vi "AI Channel Update.vi"(7 "Device Ref":T4 format="%.0x", 8 "error in (no error)":errorcluster caption="错误输入（无错误）", 11 "DIChannel":T1[](array[typedef])) -> (0 "error out":errorcluster caption="错误输出")   [LabVIEW 2013]
uses:
  <vilib>/K2Labs/HiLab API/Custom Device API/Controls/Custom Device Item Reference.ctl
  AI Param.ctl
  MeasurementType.ctl
  AI Terminal Configuration.ctl
  <vilib>/K2Labs/HiLab API/Custom Device API/Controls/Custom Device Channel.ctl
  <vilib>/K2Labs/HiLab API/Custom Device API/Controls/Custom Device Channel Dimensions.ctl
  <vilib>/K2Labs/HiLab API/Custom Device API/Controls/Custom Device Channel Type.ctl
  <vilib>/K2Labs/HiLab API/Custom Device API/Configuration/Item Properties/Set Item Property/Set Item Property(String).vi
  <vilib>/K2Labs/HiLab API/Custom Device API/Configuration/Item Properties/Set Item Property/Set Item Property(I16).vi
  <vilib>/K2Labs/HiLab API/Custom Device API/Configuration/Item Properties/Set Item Property/Set Item Property(Double).vi
  <vilib>/K2Labs/HiLab API/Custom Device API/Custom Device API Library.lvlib
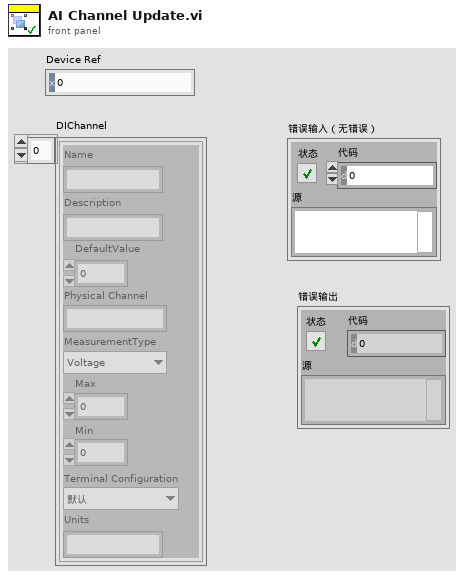
[diagram p1: front panel]
types:
  T1 = typedef "AI Param.ctl" = cluster{"Name":string, "Description":string, "DefaultValue":dbl, "Physical Channel":string, "MeasurementType":T2, "Max":dbl, "Min":dbl, "Terminal Configuration":T3, "Units":string}
  T2 = typedef "MeasurementType.ctl" = enum16{"Voltage", "Current", "More:Voltage:Custom with Excitation", "More:Current:Custom with Excitation", "Frequency", "Period", "Resistance", "Temperature:Thermocouple", "Temperature:Thermistor", "Temperature:RTD", "Temperature:Built-in Sensor", "Strain Gage"}
  T3 = typedef "AI Terminal Configuration.ctl" = enum16{"默认", "RSE", "NRSE", "差分", "伪差分"}
  T4 = typedef "Custom Device API Library.lvlib/Custom Device Item Reference.ctl" = u64
  T5 = typedef "Custom Device API Library.lvlib/Custom Device Channel.ctl" = cluster{"DefaultValue":dbl[], "Dimensions":T6, "Units":string, "Type":T7}
  T6 = typedef "Custom Device API Library.lvlib/Custom Device Channel Dimensions.ctl" = cluster{"Row":i32, "Column":i32}
  T7 = typedef "Custom Device API Library.lvlib/Custom Device Channel Type.ctl" = enum16{"Input", "Output"}
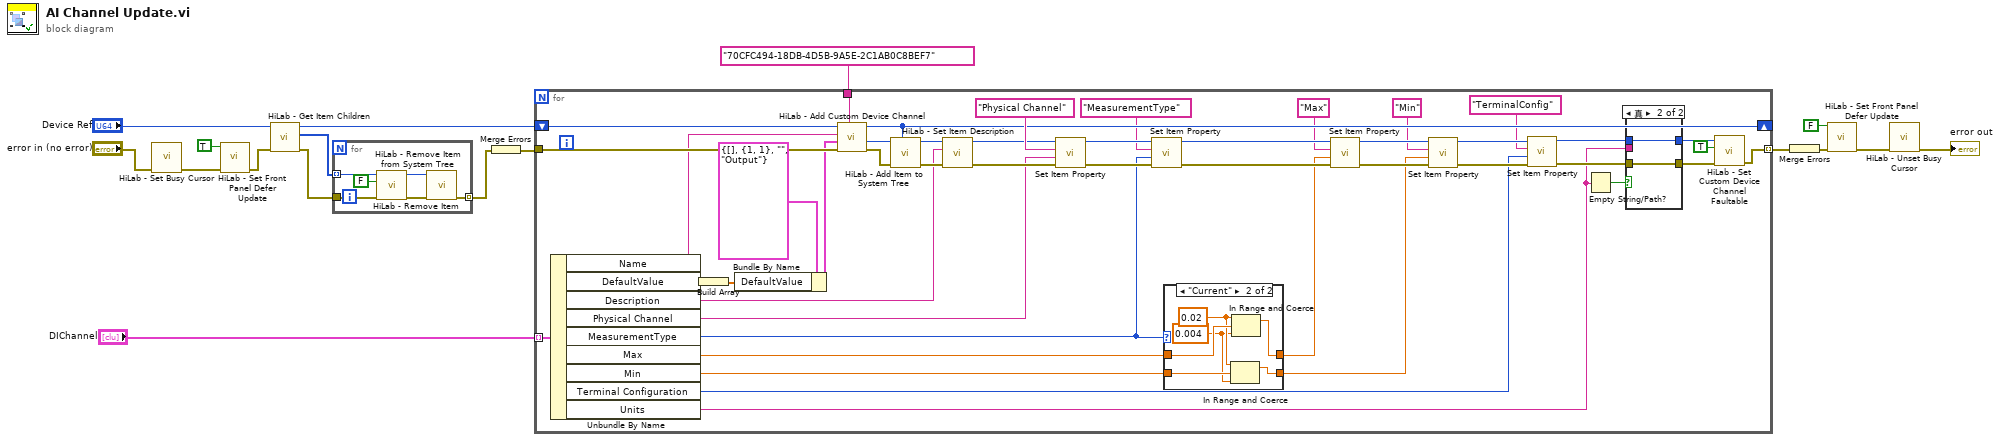
[diagram p0: block diagram]
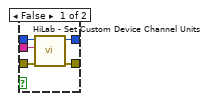
[diagram p2: hidden frame]
diagram:
  n1 = call <vilib>:"HiLab - Set Busy Cursor.vi"("error in (no error)"="error in (no error)") -> ("error out"=w15:errorcluster)  [unwired: 10 in]
  n2 = call <vilib>:"HiLab - Set Front Panel Defer Update.vi"("error in (no error)"=w15, "DeferSystemConfigurationPanUpdates(F)"=TRUE) -> ("error out"=w5:errorcluster)  [unwired: 9 in]
  n3 = call <vilib>:"HiLab - Get Item Children.vi"("error in (no error)"=w5, "Item Ref in"="Device Ref") -> ("error out"=w8:errorcluster, "Child Refs"=w7:T4[], "Item Ref out"=w3:T4)  [unwired: 6 in, 1 out]
  n4 = for {
    tunnel: w8 -> [w20]
    tunnel: [w19] -> w9 mode=indexing
    tunnel: w7 -> [w18] mode=indexing
    n5 = call <vilib>:"HiLab - Remove Item from System Tree.vi"("error in (no error)"=w20, "HighLightPreviousItem?(T)"=FALSE, "Item Ref in"=w18) -> ("error out"=w22:errorcluster, "Item Ref out"=w23:T4)  [unwired: 7 in]
    n6 = call <vilib>:"HiLab - Remove Item.vi"("error in (no error)"=w22, "Item Ref"=w23) -> ("error out"=w19:errorcluster)  [unwired: 9 in]
  }
  n7 = Merge Errors(w9) -> (w4:errorcluster)
  n8 = for {
    tunnel: w4 -> [w67]
    tunnel: [w60] -> w10 mode=indexing
    shift-right: [w62] -> _
    shift-left: w3 -> [w68]
    tunnel: "DIChannel" -> [w54] mode=indexing
    tunnel: "70CFC494-18DB-4D5B-9A5E-2C1AB0C8BEF7" ("GUID (Default Channel)") -> [w48]
    n9 = Unbundle By Name(w54) -> ("Name"=w53:string, "DefaultValue"=w50:dbl, "Description"=w51:string, "Physical Channel"=w49:string, "MeasurementType"=w38:T2, "Max"=w37:dbl, "Min"=w36:dbl, "Terminal Configuration"=w31:T3, "Units"=w25:string)
    n10 = Build Array(w50) -> (w52:dbl[])
    n11 = Bundle By Name(cluster=T5 {"DefaultValue"=[], "Dimensions"={"Row"=1, "Column"=1}, "Units"="", "Type"=enum."Output"} ("Channel"), "DefaultValue"=w52) -> (w65:T5)
    n12 = call <vilib>:"HiLab - Add Custom Device Channel.vi"("GUID (Default Channel)"=w48, "error in (no error)"=w67, "Channel"=w65, "Channel Name"=w53, "Parent Ref in"=w68) -> ("error out"=w61:errorcluster, "Channel Ref"=w63:T4, "Parent Ref out"=w62:T4)  [unwired: 3 in, 1 out]
    n13 = call <vilib>:"HiLab - Add Item to System Tree.vi"("Parent Item Ref"=w62, "error in (no error)"=w61, "Item Ref in"=w63) -> ("error out"=w55:errorcluster, "Item Ref out"=w57:T4)  [unwired: 7 in]
    n14 = call <vilib>:"HiLab - Set Item Description.vi"("error in (no error)"=w55, "Discription"=w51, "Item Ref in"=w57) -> ("error out"=w56:errorcluster, "Item Ref out"=w58:T4)  [unwired: 6 in, 1 out]
    n15 = call-poly <vilib>:"Set Item Property.vi"("error in (no error)"=w56, "Value"=w49, "Property Name"="Physical Channel", "Item Ref in"=w58) -> ("error out"=w42:errorcluster, "Item Ref out"=w43:T4)  [unwired: 5 in, 1 out]
    n16 = call-poly <vilib>:"Set Item Property.vi"("error in (no error)"=w42, "Value"=w38, "Property Name"="MeasurementType", "Item Ref in"=w43) -> ("error out"=w45:errorcluster, "Item Ref out"=w47:T4)  [unwired: 5 in, 1 out]
    n17 = case shown="\"Current\"" w38 {
      tunnel: w37 -> [w77 w82]
      tunnel: w36 -> [w76 w81]
      tunnel: [w77 w83] -> w34
      tunnel: [w76 w80] -> w35
      frame "Voltage", Default {
      }
      frame "Current" {
        w78 = 0.004 ("下限")
        w79 = 0.02 ("上限")
        n18 = In Range and Coerce(upper limit=w79, x=w81, lower limit=w78) -> (coerced(x)=w80:dbl)  [unwired: 1 out]
        n19 = In Range and Coerce(upper limit=w79, x=w82, lower limit=w78) -> (coerced(x)=w83:dbl)  [unwired: 1 out]
      }
    }
    n20 = call-poly <vilib>:"Set Item Property.vi"("error in (no error)"=w45, "Value"=w34, "Property Name"="Max", "Item Ref in"=w47) -> ("error out"=w44:errorcluster, "Item Ref out"=w46:T4)  [unwired: 5 in, 1 out]
    n21 = call-poly <vilib>:"Set Item Property.vi"("error in (no error)"=w44, "Value"=w35, "Property Name"="Min", "Item Ref in"=w46) -> ("error out"=w33:errorcluster, "Item Ref out"=w32:T4)  [unwired: 5 in, 1 out]
    n22 = call-poly <vilib>:"Set Item Property.vi"("error in (no error)"=w33, "Value"=w31, "Property Name"="TerminalConfig", "Item Ref in"=w32) -> ("error out"=w28:errorcluster, "Item Ref out"=w29:T4)  [unwired: 5 in, 1 out]
    n23 = Empty String/Path?(string/path=w25) -> (empty?=w24:bool)
    n24 = case shown="真" w24 {
      tunnel: w29 -> [w73 w75]
      tunnel: w28 -> [w72 w74]
      tunnel: [w71 w75] -> w27
      tunnel: [w70 w74] -> w26
      tunnel: w25 -> [w69 _]
      frame False {
        n25 = call <vilib>:"HiLab - Set Custom Device Channel Units.vi"("error in (no error)"=w72, "Units"=w69, "Channel Ref in"=w73) -> ("error out"=w70:errorcluster, "Channel Ref out"=w71:T4)  [unwired: 7 in]
      }
      frame True {
      }
    }
    n26 = call <vilib>:"HiLab - Set Custom Device Channel Faultable.vi"("error in (no error)"=w26, "Faultable"=TRUE, "Channel Ref in"=w27) -> ("error out"=w60:errorcluster)  [unwired: 7 in, 1 out]
  }
  n27 = Merge Errors(w10) -> (w11:errorcluster)
  n28 = call <vilib>:"HiLab - Set Front Panel Defer Update.vi"("error in (no error)"=w11, "DeferSystemConfigurationPanUpdates(F)"=FALSE) -> ("error out"=w13:errorcluster)  [unwired: 9 in]
  n29 = call <vilib>:"HiLab - Unset Busy Cursor.vi"("error in (no error)"=w13) -> ("error out"=→"error out":errorcluster)  [unwired: 10 in]
